vi "4155C VAR1 Correct Step.vi"(8 "step":dbl=2.0 format="%^.4e", 9 "stop":dbl=1.0 format="%^.4e", 10 "start":dbl format="%^.4e", 11 "sweep spacing (linear: 0)":u16(ring) items=["linear", "log 10", "log 25", "log 50"]) -> (0 "Corrected Step":dbl format="%.2f", 1 "Corrected Stop":dbl=1.0 format="%^.4e", 2 "Number of points":i32=1, 3 "dup start":dbl format="%^.4e")   [LabVIEW 2016]
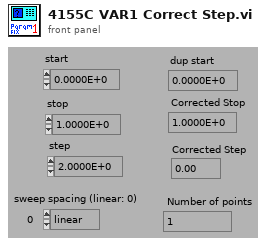
[diagram p1: front panel]
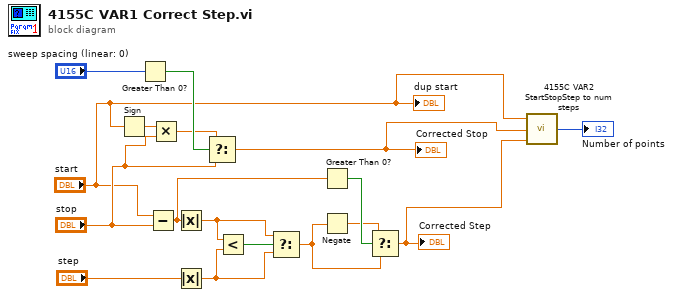
[diagram p0: block diagram]
diagram:
  n1 = Sign(1:"start") -> (0:w9:dbl)
  n2 = Greater Than 0?(x="sweep spacing (linear: 0)") -> (x > 0?=w10:bool)
  n3 = Subtract(x="start", y="stop") -> (x-y=w15:dbl)
  n4 = Multiply(x=w9, y="stop") -> (x*y=w7:dbl)
  n5 = Absolute Value(x=w15) -> (abs(x)=w6:dbl)
  n6 = Absolute Value(x="step") -> (abs(x)=w5:dbl)
  n7 = Select(t=w7, s=w10, f="stop") -> (s? t:f=w3:dbl)
  "Corrected Stop" <- w3
  n8 = Less?(x=w6, y=w5) -> (x < y?=w16:bool)
  n9 = Select(t=w6, s=w16, f=w5) -> (s? t:f=w12:dbl)
  n10 = Greater Than 0?(x=w15) -> (x > 0?=w14:bool)
  n11 = Negate(x=w12) -> (-x=w13:dbl)
  n12 = Select(t=w13, s=w14, f=w12) -> (s? t:f=w2:dbl)
  "Corrected Step" <- w2
  n13 = call "4155C VAR2 StartStopStep to num steps.vi"("step"=w2, "stop"=w3, "start"="start") -> ("Number of points"=→"Number of points":i32)  [unwired: 2 out]
  "dup start" <- "start"
